vi "Save Channel Info and Overwrite Original File.vi"(6 "Sample rate":sgl format="%.2f", 8 "error in":errorcluster, 9 "time":dbl format="%.2f", 10 "channel info":T1(array[cluster]) {"sensor sensitivity (mV/EU)" format="%.2f"; "offset" format="%.2f"; "multiplier" format="%.2f"}, 11 "refnum in":refnum<file>) -> (0 "error out":errorcluster, 3 "refnum out":refnum<file>)   [LabVIEW 2017]
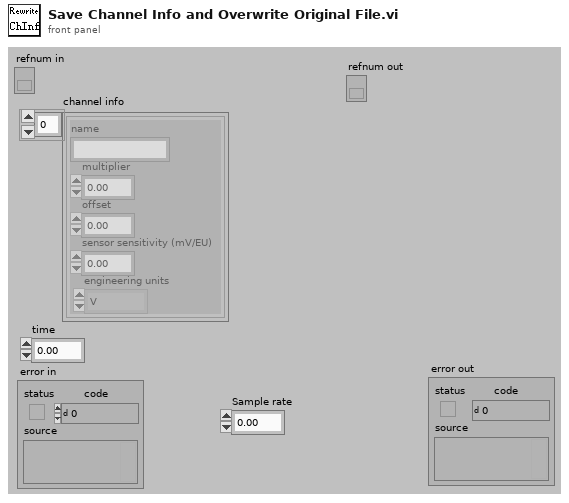
[diagram p1: front panel]
types:
  T1 = cluster{"name":string, "multiplier":sgl, "offset":sgl, "sensor sensitivity (mV/EU)":dbl, "engineering units":enum16{"custom...", "V", "Pa", "g", "m/s^2", "m/s", "m", "in/s^2", "in/s", "in"}}[]
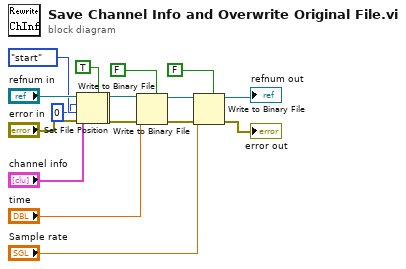
[diagram p0: block diagram]
diagram:
  n1 = Set File Position(offset (in bytes) (0)=0 ("pos offset (0)"), refnum="refnum in", from (0:start)=enum16{"start", "end", "current"}."start" ("pos mode (0:2)"), error in="error in") -> (refnum out=w4:refnum<file>, error out=w3:errorcluster)
  n2 = Write to Binary File(file (use dialog)=w4, data="channel info", error in=w3, 5:TRUE ("header (F)")) -> (refnum out=w16:refnum<file>, error out=w17:errorcluster)  [unwired: 2 in, 1 out]
  n3 = Write to Binary File(file (use dialog)=w16, data="time", error in=w17, 5:FALSE ("prepend array or string size? (T)")) -> (refnum out=w15:refnum<file>, error out=w14:errorcluster)  [unwired: 2 in, 1 out]
  n4 = Write to Binary File(file (use dialog)=w15, data="Sample rate", error in=w14, 5:FALSE ("prepend array or string size? (T)")) -> (refnum out=→"refnum out":refnum<file>, error out=→"error out":errorcluster)  [unwired: 2 in, 1 out]
